vi "Unit test-AVI save load.vi"() -> ()   [LabVIEW 2017]
uses:
  Typedefs/AVI implementation enum.ctl
  Typedefs/Channel Selector.ctl
  <userlib>/_MGI/File/MGI Windows Folder Enum.ctl
  Typedefs/Controls/AOL_Globals.ctl
  Typedefs/Imaging Protocols enum.ctl
  Typedefs/Frame Size.ctl
  Typedefs/AOL modes.ctl
  Typedefs/Plane Mode.ctl
panel:
  in  "Frame Size":T1(ring)=enum."512X512"
  in  "Frames":i32=1000
  in  "AVI mode":enum16{"AVI1 Read", "AVI2 Read"}(ring)=enum."AVI2 Read"
  out "File size (GB)":dbl format="%#.2f"
  in  "AVI mode":T2=enum."AVI2"
  out "Write speed (fps)":dbl format="%#.1f"
  out "Read speed (fps)":dbl format="%#.1f"
  out "Time to read (sec)":dbl
  out "Read error":errorcluster
  out "Stopped reading at frame #":i32
  out "Time to write (sec)":dbl
  out "Frame write loop":i32
  out "Write error":errorcluster
  out "Number of frames":i32
  out "Match":bool
  in  "base path":path
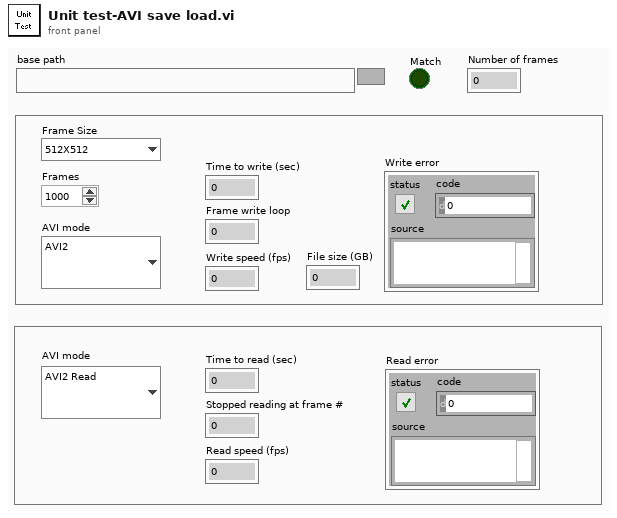
[diagram p1: front panel]
types:
  T1 = enum16{"100X100", "128X128", "200X200", "256X256", "512X512"}
  T2 = typedef "AVI implementation enum.ctl" = enum16{"AVI1", "AVI2"}
  T3 = typedef "Channel Selector.ctl" = enum16{"Red Channel", "Green Channel", "Blended"}
  T4 = typedef "MGI Windows Folder Enum.ctl" = enum32{"Desktop", "Err<Internet>", "Programs", "Err<Controls>", "Err<Printers>", "Personal (MyDocuments)", "Favorites", "Startup", "Recent", "SendTo", "Err<RecycleBin>", "StartMenu", "Err<MyDocuments>", "MyMusic", "MyVideo", "Err<0x000F>", "DesktopDirectory", "Err<Drives>", "Err<Network>", "NetHood", "Fonts", "Templates", "CommonStartMenu", "CommonPrograms", "CommonStartup", "CommonDesktopDirectory", "AppData", "PrintHood", "LocalAppData", "Err<AltStartup>", "Err<CommonAltStartup>", "CommonFavorites", "InternetCache", "Cookies", "History", "CommonAppData", "Windows", "System", "ProgramFiles", "MyPictures", "Profile", "System32", "Err<0x002A>", "ProgramFilesCommon", "Err<0x002C>", "CommonTemplates", "CommonDocuments", "CommonAdminTools", "AdminTools"}
  T5 = enum16{"Write Red AVI", "Write Green AVI", "Write AVI mode"}
  T6 = typedef "AOL_Globals.ctl" = cluster{"Imaging Protocol":T7, "Number of POI":u16, "Number of Miniscans":u16, "Number of Trials":u16, "Number of Cycles ":u64, "# Averaged Frames":u16, "Laser power (%)":u8, "Pockels":dbl, "Acquisition Length (sec)":dbl, "Fill time (us)":dbl, "POI Dwell time (us)":dbl, "Miniscan Dwell time per pixel (us)":dbl, "PMT 1":dbl, "PMT 2":dbl, "Back Apperture":dbl, "Frame Size":T8, "Center Frequency":dbl, "Field of View":dbl, "DwellTime (us)":dbl, "Wavelength (nm)":dbl, "Zoom":dbl, "AOL Z":dbl, "AOL Mode":T9, "GridXY":dbl, "GridZ":dbl, "TriggerPeriod (sec)":dbl, "Number of Pixels in Miniscan":u16, "Experiment folder path":path, "X centre":dbl, "Y centre":dbl, "Angle (degrees)":dbl, "Plane Mode":T10, "Threshold":u16[], "Regenerate Chirps":bool, "Rectangle ROI length (pixels)":u16, "Rectangle ROI height (pixels)":u16, "AOD fill":u16, "StartupDelay":i32, "Samples Wait after Trigger":u16, "Slip Cycle":u32, "Add Cycle":bool}
  T7 = typedef "Imaging Protocols enum.ctl" = enum16{"AOL Z-Stack", "Motor Z Stack", "Functional Acquisition", "Single Plane Acquisition", "Volume Acquisition", "Live Imaging", "Live Plane Imaging", "Live Volume Imaging"}
  T8 = typedef "Frame Size.ctl" = u16
  T9 = typedef "AOL modes.ctl" = enum16{"Raster", "Structural", "Pointing", "Mini Scan", "Alignment"}
  T10 = typedef "Plane Mode.ctl" = u16
  T11 = typedef "AVI Refs cluster.ctl" = cluster{"AVI2 path":path, "AVI 2 Refnum":T12, "New Image":T13, "error out":errorcluster, "Avi 1 Refnum":T14}
  T12 = typedef "IMAQ AVI2 Refnum.ctl" = refnum<k20>
  T13 = typedef "IMAQ Image.ctl" = refnum<image>
  T14 = typedef "AviRefnum.ctl" = refnum<k1>
  T15 = typedef "Image Type" = u32
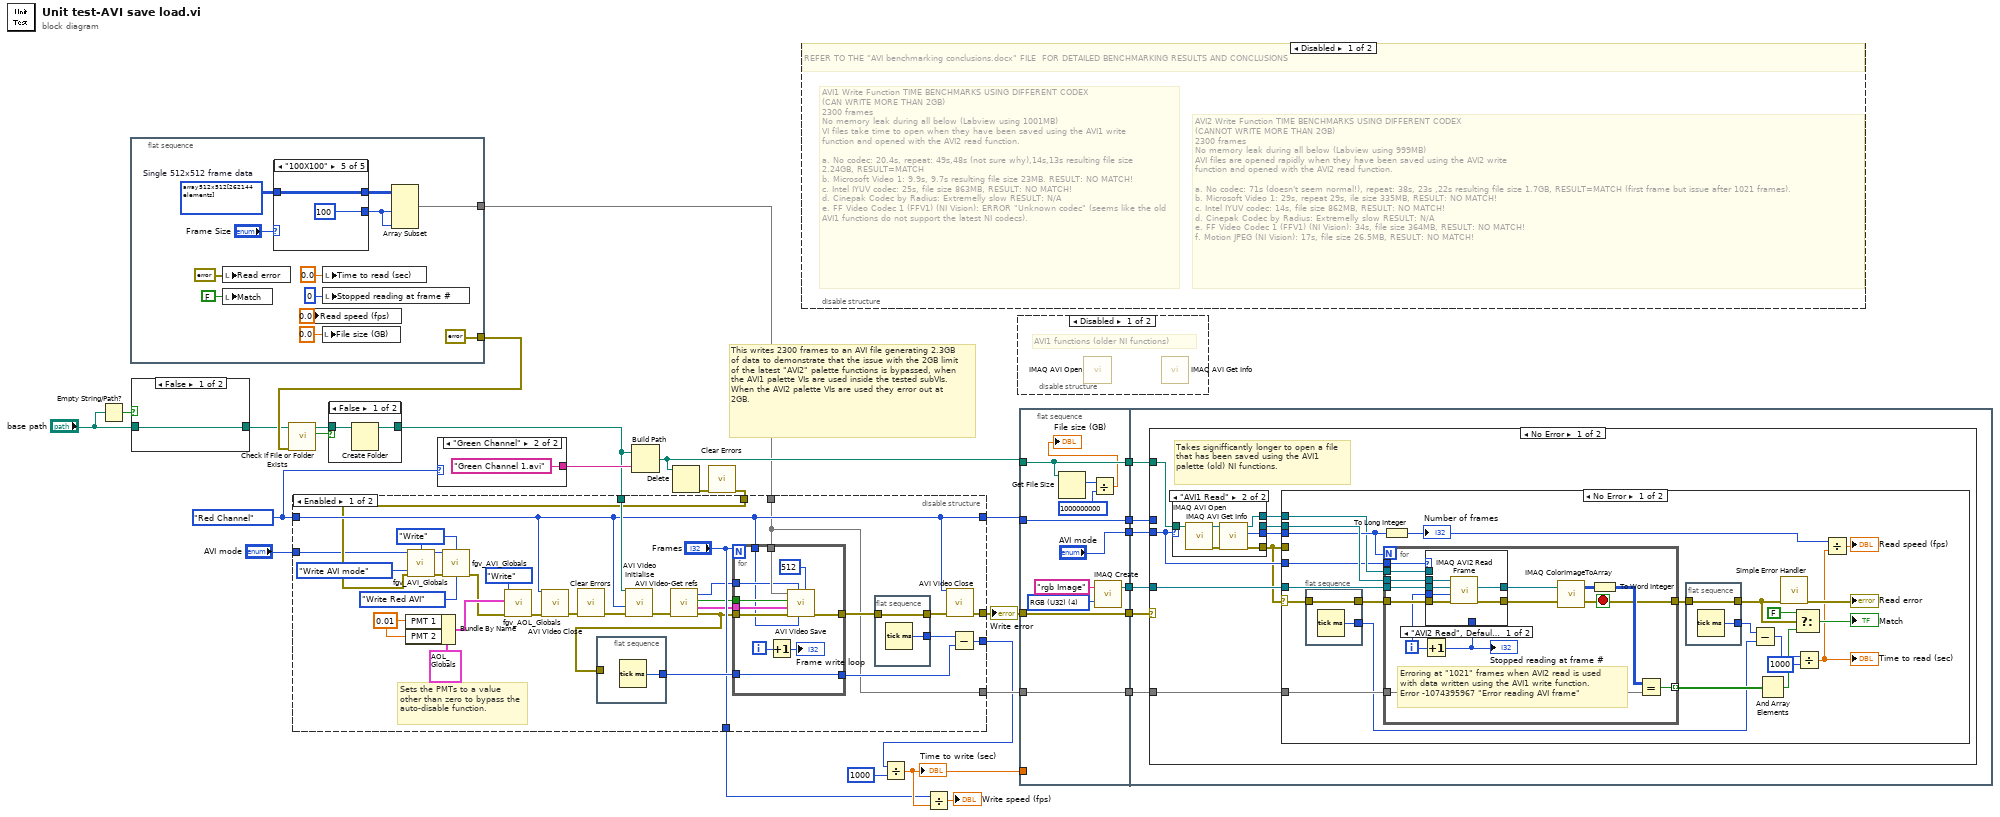
[diagram p0: block diagram]
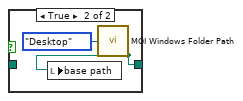
[diagram p3: hidden frame]
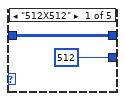
[diagram p4: hidden frame]
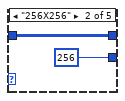
[diagram p5: hidden frame]
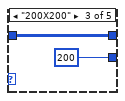
[diagram p6: hidden frame]
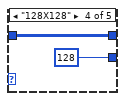
[diagram p7: hidden frame]
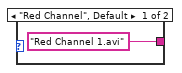
[diagram p8: hidden frame]
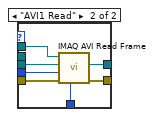
[diagram p12: hidden frame]
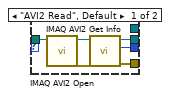
[diagram p14: hidden frame]
diagram:
  w18 = Channel_Selector."Red Channel" ("Channel")
  # "This writes 2300 frames to an AVI file generating 2.3GB of data to demonstrate that the issue with the 2GB limit of the latest \"AVI2\" palette functions is bypassed, when the AVI1 palette VIs are used inside the tested subVIs. When the AVI2 palette VIs are used they error out at 2GB."
  n1 = Empty String/Path?(string/path="base path") -> (empty?=w6:bool)
  n2 = flat-sequence {
    tunnel: [errorcluster {"status"=FALSE, "code"=0, "source"=""} ("error out")] -> w13
    tunnel: [w29] -> w3
    frame #0 {
      w32 = i16[][] array512x512[262144 elements]  # Single 512x512 frame data
      n3 = local write "Read error"(errorcluster {"status"=FALSE, "code"=0, "source"=""} ("error out")) -> ()
      n4 = local write "Match"(FALSE ("Match")) -> ()
      n5 = case shown="\"100X100\"" "Frame Size" {
        tunnel: [w42 w44 w46 w48 w50] -> w31
        tunnel: w32 -> [w42 w44 w46 w48 w50]
        tunnel: [512 ("length") 256 ("length") 200 ("length") 128 ("length") 100 ("length")] -> w33
        frame "512X512" {
        }
        frame "256X256" {
        }
        frame "200X200" {
        }
        frame "128X128" {
        }
        frame "100X100" {
        }
      }
      n6 = local write "Read speed (fps)"(0.0 ("Read FPS")) -> ()
      n7 = local write "File size (GB)"(0.0 ("File size (GB)")) -> ()
      n8 = local write "Time to read (sec)"(0.0 ("Time to read (sec)")) -> ()
      n9 = local write "Stopped reading at frame #"(0 ("Stopped reading at frame #")) -> ()
      n10 = Array Subset(array=w31, length (row)=w33, length (col)=w33) -> (w29:i16[][])  [unwired: 2 in]
    }
  }
  n11 = case shown="False" w6 {
    tunnel: "base path" -> [w51 _]
    tunnel: [w51 w52] -> w4
    frame False {
    }
    frame True {
      n12 = call <userlib>:"MGI Windows Folder Path.vi"("Windows Folder"=MGI_Windows_Folder_Enum."Desktop") -> ("Path"=w52:path)
      n13 = local write "base path"(w52) -> ()
    }
  }
  n14 = call <vilib>:"Check if File or Folder Exists.vi"("error in (no error)"=w13, "path"=w4) -> ("file or folder exists?"=w21:bool, "dup path"=w22:path)  [unwired: 7 in, 1 out]
  n15 = case shown="False" w21 {
    tunnel: [w55 w56] -> w19
    tunnel: w22 -> [w54 w56]
    frame False {
      n16 = Create Folder(path (use dialog)=w54) -> (created path=w55:path)  [unwired: 2 in, 2 out]
    }
    frame True {
    }
  }
  n17 = case shown="\"Green Channel\"" w18 {
    tunnel: ["Red Channel 1.avi" ("name or relative path") "Green Channel 1.avi" ("name or relative path")] -> w20
    frame "Red Channel", Default {
    }
    frame "Green Channel" {
    }
  }
  n18 = Build Path(base path=w19, name or relative path=w20) -> (appended path=w17:path)
  n19 = Delete(path (use dialog)=w17) -> (error out=w16:errorcluster)  [unwired: 4 in, 2 out]
  n20 = call <vilib>:"Clear Errors.vi"("error in (no error)"=w16) -> ("error out"=w15:errorcluster)  [unwired: 5 in, 1 out]
  n21 = disable-structure shown="Enabled" {
    disable-tunnel: w19 -> [w88 _]
    disable-tunnel: [w87 _] -> w25
    disable-tunnel: [w81 _] -> w1
    disable-tunnel: [w64 w103] -> w28
    disable-tunnel: [w72 _] -> w27
    disable-tunnel: w18 -> [w72 _]
    disable-tunnel: w15 -> [w71 _]
    disable-tunnel: "AVI mode" -> [w61 _]
    disable-tunnel: ["Frames" _] -> w2
    disable-tunnel: w3 -> [w64 _]
    frame Enabled {
      w60 = enum16{"Intialize", "Write", "Read", "Clear"}."Write" ("Function")
      w77 = 0.01 ("PMT 1")
      # "Sets the PMTs to a value other than zero to bypass the auto-disable function."
      n22 = Bundle By Name(cluster=T6 {"Imaging Protocol"=enum."AOL Z-Stack", "Number of POI"=0, "Number of Miniscans"=0, "Number of Trials"=0, "Number of Cycles "=0, "# Averaged Frames"=0, "Laser power (%)"=0, "Pockels"=0.0, "Acquisition Length (sec)"=0.0, "Fill time (us)"=0.0, "POI Dwell time (us)"=0.0, "Miniscan Dwell time per pixel (us)"=0.0, "PMT 1"=0.0, "PMT 2"=0.0, "Back Apperture"=200.0, "Frame Size"=0, "Center Frequency"=0.0, "Field of View"=0.0, "DwellTime (us)"=0.0, "Wavelength (nm)"=0.0, "Zoom"=0.0, "AOL Z"=0.0, "AOL Mode"=enum."Raster", "GridXY"=0.0, "GridZ"=0.0, "TriggerPeriod (sec)"=0.0, "Number of Pixels in Miniscan"=0, "Experiment folder path"=path "", "X centre"=0.0, "Y centre"=0.0, "Angle (degrees)"=0.0, "Plane Mode"=0, "Threshold"=[], "Regenerate Chirps"=FALSE, "Rectangle ROI length (pixels)"=0, "Rectangle ROI height (pixels)"=0, "AOD fill"=0, "StartupDelay"=0, "Samples Wait after Trigger"=0, "Slip Cycle"=0, "Add Cycle"=FALSE} ("AOL_Globals"), "PMT 1"=w77, "PMT 2"=w77) -> (w78:T6)
      n23 = call "fgv_AVI_Globals.vi"("AVI mode"=w61, "Function"=w60, "error in (no error)"=w71, "\"Write\" sub function"=T5."Write AVI mode" ("\"Write\" sub function")) -> ("error out"=w63:errorcluster)  [unwired: 8 in, 3 out]
      n24 = call "fgv_AVI_Globals.vi"("AVI mode"=w61, "Function"=w60, "error in (no error)"=w63, "\"Write\" sub function"=T5."Write Red AVI" ("\"Write\" sub function")) -> ("error out"=w62:errorcluster)  [unwired: 8 in, 3 out]
      n25 = call "fgv_AOL_Globals.vi"("error in (no error)"=w62, "AOL_Globals"=w78, "Function"=enum16{"Intialize", "Write", "Read", "Clear"}."Write") -> ("error out"=w74:errorcluster)  [unwired: 7 in, 1 out]
      n26 = call "AVI Video Close.vi"("error in (no error)"=w74, "Channel"=w72) -> ("error out"=w79:errorcluster)  [unwired: 9 in]
      n27 = call <vilib>:"Clear Errors.vi"("error in (no error)"=w79) -> ("error out"=w80:errorcluster)  [unwired: 5 in, 1 out]
      n28 = flat-sequence {
        tunnel: [w89] -> w86
        tunnel: w68 -> [_]
        frame #0 {
          n29 = Tick Count (ms)() -> (millisecond timer value=w89:u32)
        }
      }
      n30 = call "AVI Video Initialise.vi"("error in (no error)"=w80, "Channel"=w72, "Timelapse folder path"=w88) -> ("error out"=w69:errorcluster)  [unwired: 8 in]
      n31 = call "AVI Video-Get refs.vi"("error in (no error)"=w69) -> ("error out"=w68:errorcluster, "AVI mode"=w65:T2, "Red AVI"=w66:T11, "Red PMT is ON"=w67:bool)  [unwired: 4 in, 3 out]
      n32 = for {
        N: "Frames" -> [_]
        tunnel: w72 -> [w93]
        tunnel: w64 -> [w97]
        tunnel: [w101] -> w85
        tunnel: w68 -> [w102]
        tunnel: w86 -> [w99]
        tunnel: [w99] -> w82
        tunnel: w65 -> [w96]
        tunnel: w67 -> [w95]
        tunnel: w66 -> [w94]
        i -> [w100]
        n33 = Increment(x=w100) -> (x+1=→"Frame write loop":i32)
        n34 = call "AVI Video Save.vi"("Frame Size"=u32 512, "Channel"=w93, "AVI mode"=w96, "error in (no error)"=w102, "AVI cluster"=w94, "PMT is ON?"=w95, "Image Pixels"=w97) -> ("error out"=w101:errorcluster)  [unwired: 3 in, 1 out]
      }
      n35 = flat-sequence {
        tunnel: w85 -> [w91]
        tunnel: [w91] -> w84
        tunnel: [w90] -> w83
        frame #0 {
          n36 = Tick Count (ms)() -> (millisecond timer value=w90:u32)
        }
      }
      n37 = call "AVI Video Close.vi"("error in (no error)"=w84, "Channel"=w72) -> ("error out"=w87:errorcluster)  [unwired: 9 in]
      n38 = Subtract(x=w83, y=w82) -> (x-y=w81:u32)
    }
    frame Disabled {
    }
  }
  "Write error" <- w25
  n39 = disable-structure shown="Disabled" {
    frame Disabled {
      # "AVI2 Write Function TIME BENCHMARKS USING DIFFERENT CODEX \n(CANNOT WRITE MORE THAN 2GB)\n2300 frames\nNo memory leak during all below (Labview using 999MB)\nAVI files are opened rapidly when they have been saved using the AVI2 write \nfunction and opened with the AVI2 read function.\n\na. No codec: 71s (doesn't seem normal!), repeat: 38s, 23s ,22s resulting file size 1.7GB, RESULT=MATCH (first frame but issue after 1021 frames).\nb. Microsoft Video 1: 29s, repeat 29s, ile size 335MB, RESULT: NO MATCH!\nc. Intel IYUV codec: 14s, file size 862MB, RESULT: NO MATCH!\nd. Cinepak Codec by Radius: Extremelly slow RESULT: N/A\ne. FF Video Codec 1 (FFV1) (NI Vision): 34s, file size 364MB, RESULT: NO MATCH!\nf. Motion JPEG (NI Vision): 17s, file size 26.5MB, RESULT: NO MATCH!"
      # "AVI1 Write Function TIME BENCHMARKS USING DIFFERENT CODEX\n(CAN WRITE MORE THAN 2GB)\n2300 frames\nNo memory leak during all below (Labview using 1001MB)\nVI files take time to open when they have been saved using the AVI1 write \nfunction and opened with the AVI2 read function.\n\na. No codec: 20.4s, repeat: 49s,48s (not sure why),14s,13s resulting file size 2.24GB, RESULT=MATCH\nb. Microsoft Video 1: 9.9s, 9.7s resulting file size 23MB. RESULT: NO MATCH!\nc. Intel IYUV codec: 25s, file size 863MB, RESULT: NO MATCH!\nd. Cinepak Codec by Radius: Extremelly slow RESULT: N/A\ne. FF Video Codec 1 (FFV1) (NI Vision): ERROR \"Unknown codec\" (seems like the old AVI1 functions do not support the latest NI codecs)."
      # "REFER TO THE \"AVI benchmarking conclusions.docx\" FILE  FOR DETAILED BENCHMARKING RESULTS AND CONCLUSIONS"
    }
    frame Enabled {
      # "REFER TO THE \"AVI benchmarking conclusions.docx\" FILE  FOR DETAILED BENCHMARKING RESULTS AND CONCLUSIONS"
    }
  }
  n40 = Divide(x=w1, y=u32 1000) -> (x/y=w23:dbl)
  "Time to write (sec)" <- w23
  n41 = Divide(x=w2, y=w23) -> (x/y=→"Write speed (fps)":dbl)
  n42 = disable-structure shown="Disabled" {
    frame Disabled {
      # "AVI1 functions (older NI functions)"
      n43 = call "IMAQ AVI Open"() -> ()  [unwired: 10 in, 2 out]
      n44 = call "IMAQ AVI Get Info"() -> ()  [unwired: 7 in, 5 out]
    }
    frame Enabled {
    }
  }
  n45 = flat-sequence {
    tunnel: w17 -> [w109]
    tunnel: w23 -> [_]
    tunnel: w27 -> [w112]
    tunnel: w28 -> [w113]
    tunnel: w25 -> [w114]
    tunnel: [w114] -> w12
    tunnel: [w113] -> w11
    tunnel: [w112] -> w10
    tunnel: [w109] -> w9
    tunnel: [w106] -> w8
    tunnel: ["AVI mode"] -> w7
    tunnel: w12 -> [w118]
    tunnel: w11 -> [w120]
    tunnel: w10 -> [w119]
    tunnel: w9 -> [w117]
    tunnel: w8 -> [w116]
    tunnel: w7 -> [w115]
    frame #0 {
      w107 = T15 4 items=["Grayscale (U8)", "Grayscale (I16)", "Grayscale (SGL)", "Complex (CSG)", "RGB (U32)", "HSL (U32)", "RGB (U64)", "Grayscale (U16)"] ("Image Type")
      n46 = Get File Size(file=w109) -> (size (in bytes)=w110:i64)  [unwired: 1 in, 2 out]
      n47 = Divide(x=w110, y=i64 1000000000) -> (x/y=→"File size (GB)":dbl)
      n48 = call "IMAQ Create"("Image Name"="rgb Image", "Image Type"=w107) -> ("New Image"=w106:T13)  [unwired: 2 in, 2 out]
    }
    frame #1 {
      n49 = case shown="No Error" w118 {
        tunnel: w120 -> [w127 _]
        tunnel: w119 -> [_ _]
        tunnel: w117 -> [w124 _]
        tunnel: w115 -> [w123 _]
        tunnel: w116 -> [w122 _]
        frame No Error {
          # "Takes signifficantly longer to open a file that has been saved using the AVI1 palette (old) NI functions."
          n50 = case shown="\"AVI1 Read\"" w123 {
            tunnel: [w182 _] -> w128
            tunnel: [w187 w193] -> w126
            tunnel: [_ w188] -> w125
            tunnel: [w186 w192] -> w121
            tunnel: w124 -> [w185 w191]
            frame "AVI2 Read", Default {
              n51 = call "IMAQ AVI2 Open"("AVI File Path"=w185) -> ("error out"=w183:errorcluster, "AVI Refnum"=w184:T12)  [unwired: 9 in]
              n52 = call "IMAQ AVI2 Get Info"("error in (no error)"=w183, "AVI Refnum"=w184) -> ("error out"=w186:errorcluster, "Number of Frames"=w187:u32, "AVI Refnum (duplicate)"=w182:T12)  [unwired: 5 in, 2 out]
            }
            frame "AVI1 Read" {
              n53 = call "IMAQ AVI Open"("AVI Path"=w191) -> ("error out"=w189:errorcluster, "Avi Refnum"=w190:T14)  [unwired: 9 in]
              n54 = call "IMAQ AVI Get Info"("error in (no error)"=w189, "Avi Refnum"=w190) -> ("error out"=w192:errorcluster, "Number of Frames"=w193:u32, "Avi Refnum (duplicate)"=w188:T14)  [unwired: 5 in, 2 out]
            }
          }
          n55 = case shown="No Error" w121 {
            selector: w121 -> [w129 _]
            tunnel: w128 -> [w150 _]
            tunnel: w127 -> [w149 _]
            tunnel: w126 -> [w148 _]
            tunnel: w125 -> [w143 _]
            tunnel: w121 -> [_ _]
            tunnel: w123 -> [w131 _]
            tunnel: w122 -> [w130 _]
            frame No Error {
              n56 = flat-sequence {
                tunnel: w129 -> [w154]
                tunnel: [w154] -> w141
                tunnel: [w153] -> w137
                frame #0 {
                  n57 = Tick Count (ms)() -> (millisecond timer value=w153:u32)
                }
              }
              n58 = To Long Integer(number=w148) -> (32bit integer=w134:i32)
              "Number of frames" <- w134
              n59 = for {
                N: w148 -> [_]
                tunnel: w150 -> [w167]
                tunnel: w141 -> [w166]
                tunnel: w149 -> [w164]
                tunnel: w130 -> [w163]
                tunnel: [w160] -> w147 mode=indexing
                tunnel: [w158] -> w140
                tunnel: w143 -> [w157]
                tunnel: w131 -> [w155]
                i -> [w161]
                stop <- w158 stop-if-true
                # "Erroring at \"1021\" frames when AVI2 read is used \nwith data written using the AVI1 write function.\nError -1074395967 \"Error reading AVI frame\""
                n60 = Increment(x=w161) -> (x+1=w156:i32)
                "Stopped reading at frame #" <- w156
                n61 = case shown="\"AVI2 Read\", Default" w155 {
                  tunnel: [w174 w181] -> w168
                  tunnel: w167 -> [w173 _]
                  tunnel: w166 -> [w172 w180]
                  tunnel: w163 -> [w171 w179]
                  tunnel: w161 -> [w170 w178]
                  tunnel: [w169 w177] -> w159
                  tunnel: w157 -> [_ w176]
                  tunnel: w156 -> [_ w175]
                  frame "AVI2 Read", Default {
                    n62 = call "IMAQ AVI2 Read Frame"("error in (no error)"=w172, "Frame Number"=w170, "Image"=w171, "AVI Refnum"=w173) -> ("error out"=w169:errorcluster, "Image Out"=w174:T13)  [unwired: 5 in, 1 out]
                  }
                  frame "AVI1 Read" {
                    n63 = call "IMAQ AVI Read Frame"("Frame Read Lookahead"=w175, "error in (no error)"=w180, "Frame Number"=w178, "Image"=w179, "Avi Refnum"=w176) -> ("error out"=w177:errorcluster, "Image Out"=w181:T13)  [unwired: 3 in, 2 out]
                  }
                }
                n64 = call "IMAQ ColorImageToArray"("Image"=w168, "error in (no error)"=w159) -> ("Image Pixels (U32)"=w165:u32[][], "error out"=w158:errorcluster)  [unwired: 1 in, 2 out]
                n65 = To Word Integer(number=w165) -> (16bit integer=w162:i16[][])
                n66 = Equal?(x=w162, y=w164) -> (x = y?=w160:bool)
              }
              n67 = flat-sequence {
                tunnel: w140 -> [w152]
                tunnel: [w152] -> w139
                tunnel: [w151] -> w138
                frame #0 {
                  n68 = Tick Count (ms)() -> (millisecond timer value=w151:u32)
                }
              }
              n69 = Subtract(x=w138, y=w137) -> (x-y=w136:u32)
              n70 = And Array Elements(Boolean array=w147) -> (logical AND=w145:bool)
              n71 = call <vilib>:"Simple Error Handler.vi"("error in (no error)"=w139) -> ("error out"=→"Read error":errorcluster)  [unwired: 4 in, 4 out]
              n72 = Select(t=FALSE ("Match"), s=w139, f=w145) -> (s? t:f=→"Match":bool)
              n73 = Divide(x=w136, y=u32 1000) -> (x/y=w133:dbl)
              "Time to read (sec)" <- w133
              n74 = Divide(x=w134, y=w133) -> (x/y=→"Read speed (fps)":dbl)
            }
            frame Error {
            }
          }
        }
        frame Error {
        }
      }
    }
  }
